vi "Do Something Else and Wait for Reply.vi"(6 "wait for reply (T)":bool=TRUE, 8 "error in":errorcluster, 9 "X":dbl, 10 "Do Something Else Message":string, 11 "Module ID":i32=-1) -> (0 "error out":errorcluster, 1 "timed out?":bool, 3 "Value":dbl)   [LabVIEW 2025, in "My Cloneable Module.lvlib"]
doc: "Send the Do Something Else request to the Module's Main.vi.\n_____\nBased on DQMH Dev Tools: Project Template 7.1.0.1503."
uses:
  My Cloneable Module.lvlib
  Do Something Else and Wait for Reply Argument--cluster.ctl
  Do Something Else and Wait (Reply Payload)--cluster.ctl
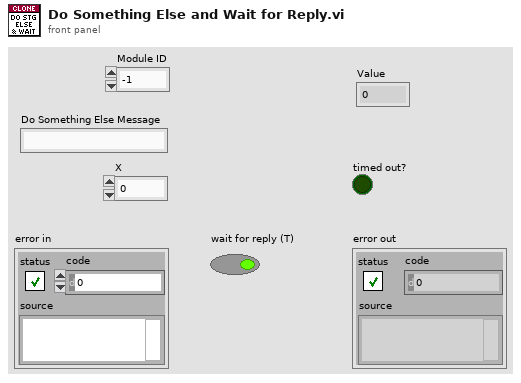
[diagram p1: front panel]
types:
  T1 = typedef "My Cloneable Module.lvlib/Request Events--cluster.ctl" = cluster{"Stop Module":refnum<user-event>, "Do Something":refnum<user-event>, "Do Something Else":refnum<user-event>, "Do Something Else and Wait for Reply":refnum<user-event>, "Show Panel":refnum<user-event>, "Hide Panel":refnum<user-event>, "Show Diagram":refnum<user-event>, "Get Module Execution Status":refnum<user-event>}
  T2 = typedef "My Cloneable Module.lvlib/Do Something Else and Wait for Reply Argument--cluster.ctl" = cluster{"Module ID":i32, "Do Something Else Msg":string, "X":dbl, "Wait Notifier":refnum<notifier>, "wait for reply":bool}
  T3 = typedef "My Cloneable Module.lvlib/Do Something Else and Wait (Reply Payload)--cluster.ctl" = cluster{"Value":dbl, "error":errorcluster, "Module ID":i32}
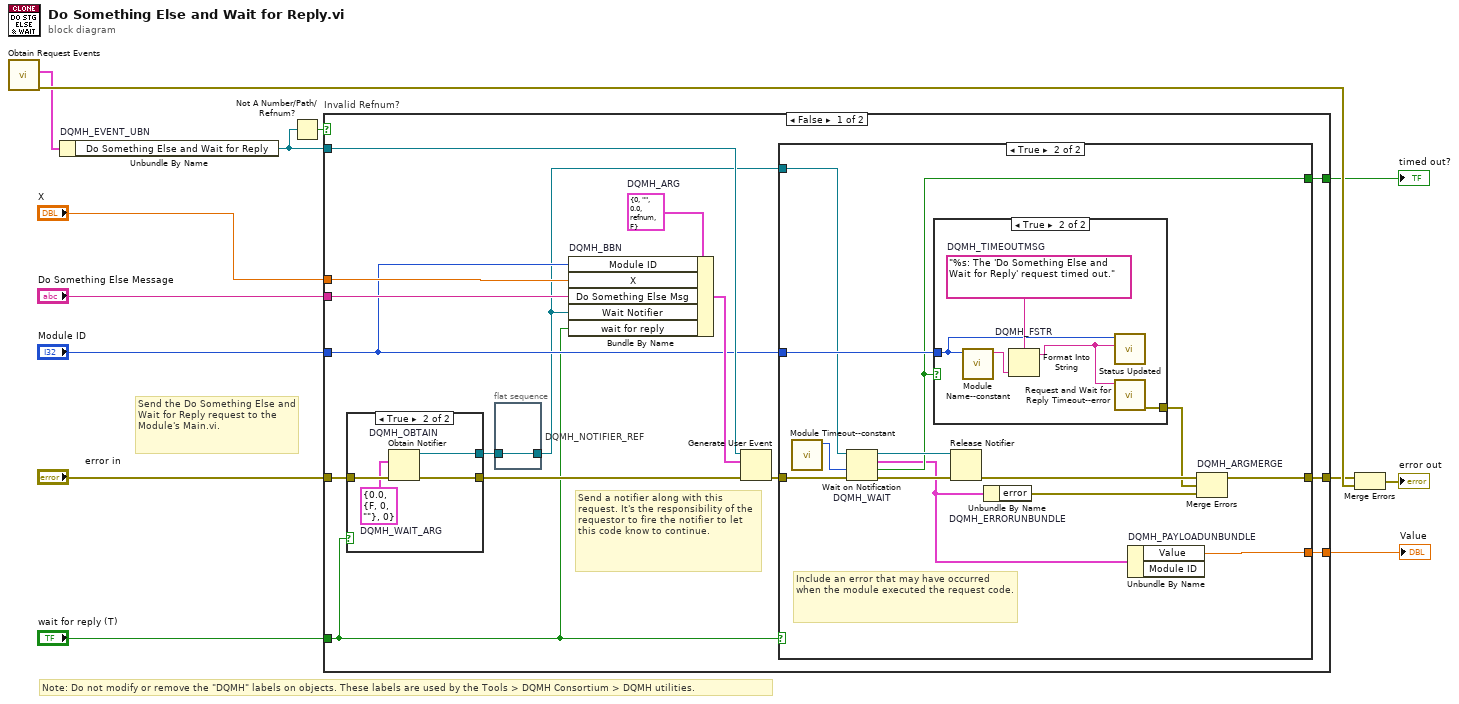
[diagram p0: block diagram]
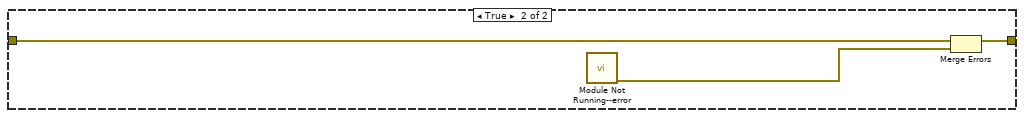
[diagram p5: hidden frame]
diagram:
  # "Note: Do not modify or remove the \"DQMH\" labels on objects. These labels are used by the Tools > DQMH Consortium > DQMH utilities."
  # "Send the Do Something Else and Wait for Reply request to the Module's Main.vi."
  n1 = call "Obtain Request Events.vi"() -> ("error out"=w12:errorcluster, "My Cloneable Module Request Events"=w11:T1)  [unwired: 10 in]
  n2 = Unbundle By Name "DQMH_EVENT_UBN"(w11) -> ("Do Something Else and Wait for Reply"=w9:refnum<user-event>)
  n3 = Not A Number/Path/Refnum?(number/path/refnum=w9) -> (NaN/Path/Refnum?=w10:bool)
  n4 = case "Invalid Refnum?" shown="False" w10 {
    tunnel: [w18 w55] -> w5
    tunnel: "X" -> [w25 _]
    tunnel: "Do Something Else Message" -> [w24 _]
    tunnel: "error in" -> [w23 w54]
    tunnel: w9 -> [w22 _]
    tunnel: "Module ID" -> [w20 _]
    tunnel: [w19 _] -> w3
    tunnel: [w17 _] -> w1
    tunnel: "wait for reply (T)" -> [w14 _]
    frame False {
      w21 = T2 {"Module ID"=0, "Do Something Else Msg"="", "X"=0.0, "Wait Notifier"=refnum, "wait for reply"=FALSE}  # DQMH_ARG
      # "Send a notifier along with this request. It's the responsibility of the requestor to fire the notifier to let this code know to continue."
      n5 = case shown="True" w14 {
        tunnel: [w49 w53] -> w26
        tunnel: [_ w52] -> w16
        tunnel: w23 -> [w49 w51]
        frame False {
        }
        frame True {
          w50 = T3 {"Value"=0.0, "error"={"status"=FALSE, "code"=0, "source"=""}, "Module ID"=0}  # DQMH_WAIT_ARG
          n6 = Obtain Notifier "DQMH_OBTAIN"(notification data type=w50, error in (no error)=w51) -> (notifier out=w52:refnum<notifier>, error out=w53:errorcluster)  [unwired: 2 in, 1 out]
        }
      }
      n7 = flat-sequence "DQMH_NOTIFIER_REF" {
        tunnel: w16 -> [w48]
        tunnel: [w48] -> w15
        frame #0 {
        }
      }
      n8 = Bundle By Name "DQMH_BBN"(cluster=w21, "Module ID"=w20, "X"=w25, "Do Something Else Msg"=w24, "Wait Notifier"=w15, "wait for reply"=w14) -> (w27:T2)
      n9 = Generate User Event(user event=w22, event data cluster=w27, error in=w26) -> (error out=w28:errorcluster)  [unwired: 1 in, 1 out]
      n10 = case shown="True" w14 {
        tunnel: w28 -> [w29 w41]
        tunnel: w20 -> [_ w37]
        tunnel: [_ w36] -> w19
        tunnel: [w29 w35] -> w18
        tunnel: [_ w30] -> w17
        tunnel: w15 -> [_ w34]
        frame False {
        }
        frame True {
          # "Include an error that may have occurred when the module executed the request code."
          n11 = call "Module Timeout--constant.vi"() -> ("Module Timeout"=w40:i32)  [unwired: 11 in]
          n12 = Wait on Notification "DQMH_WAIT"(notifier=w34, timeout in ms (-1)=w40, error in (no error)=w41) -> (notifier out=w39:refnum<notifier>, notification=w31:T3, timed out?=w36:bool, error out=w42:errorcluster)  [unwired: 1 in]
          n13 = case shown="True" w36 {
            tunnel: w37 -> [_ w45]
            tunnel: [_ w43] -> w32
            frame False {
            }
            frame True {
              w46 = "%s: The 'Do Something Else and Wait for Reply' request timed out."  # DQMH_TIMEOUTMSG
              n14 = call "Module Name--constant.vi"("Module ID"=w45) -> ("Module Name"=w47:string)  [unwired: 10 in]
              n15 = Format Into String "DQMH_FSTR"(format string=w46, w47) -> (resulting string=w44:string)  [unwired: 2 in, 1 out]
              n16 = call "Status Updated.vi"("Status"=w44, "Module ID"=w45) -> ()  [unwired: 9 in, 1 out]
              n17 = call "Request and Wait for Reply Timeout--error.vi"("Error Message"=w44) -> ("error out"=w43:errorcluster)  [unwired: 10 in]
            }
          }
          n18 = Release Notifier(notifier=w39, error in (no error)=w42) -> (error out=w38:errorcluster)  [unwired: 1 in, 2 out]
          n19 = Unbundle By Name "DQMH_ERRORUNBUNDLE"(w31) -> ("error"=w33:errorcluster)
          n20 = Unbundle By Name "DQMH_PAYLOADUNBUNDLE"(w31) -> ("Value"=w30:dbl)  [unwired: 1 out]
          n21 = Merge Errors "DQMH_ARGMERGE"(w38, w32, w33) -> (w35:errorcluster)
        }
      }
    }
    frame True {
      n22 = call "Module Not Running--error.vi"() -> ("error out"=w56:errorcluster)  [unwired: 11 in]
      n23 = Merge Errors(w54, w56) -> (w55:errorcluster)
    }
  }
  "timed out?" <- w3
  "Value" <- w1
  n24 = Merge Errors(w5, w12) -> (→"error out":errorcluster)
